vi "GT Helix ZXCY.vi"(0 "cardNum":i16, 1 "crd":i16, 2 "x":i32, 3 "y":i32, 4 "z":i32, 5 "zCenter":dbl, 6 "xCenter":dbl, 7 "error in (no error)":errorcluster caption="错误输入（无错误）", 8 "circleDir":i16, 9 "synVel":dbl, 10 "synAcc":dbl, 11 "velEnd":dbl, 12 "fifo":i16) -> (20 "function return":i16, 27 "error out":errorcluster caption="错误输出")   [LabVIEW 2014, in "gts.lvlib"]
doc: "GT_API GT_HelixZXCY(short cardNum,short crd,long x,long y,long z,double zCenter,double xCenter,short circleDir,double synVel,double synAcc,double velEnd=0,short fifo=0);"
uses:
  gts.lvlib
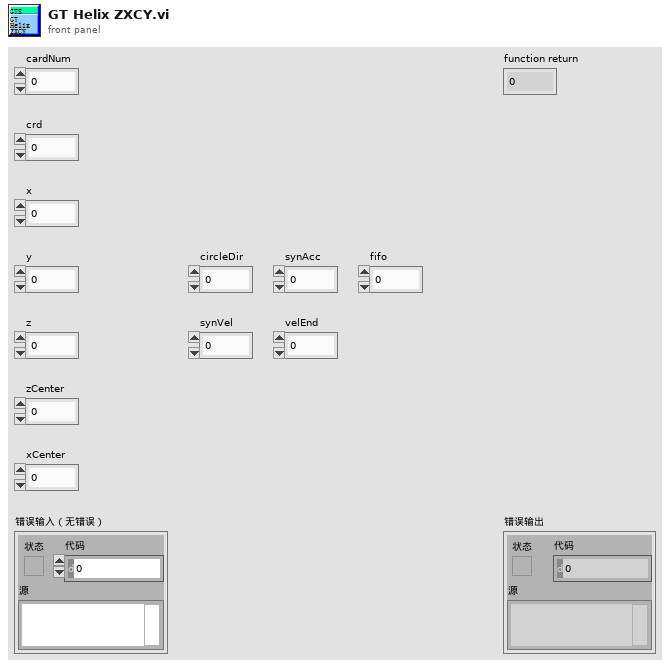
[diagram p1: front panel]
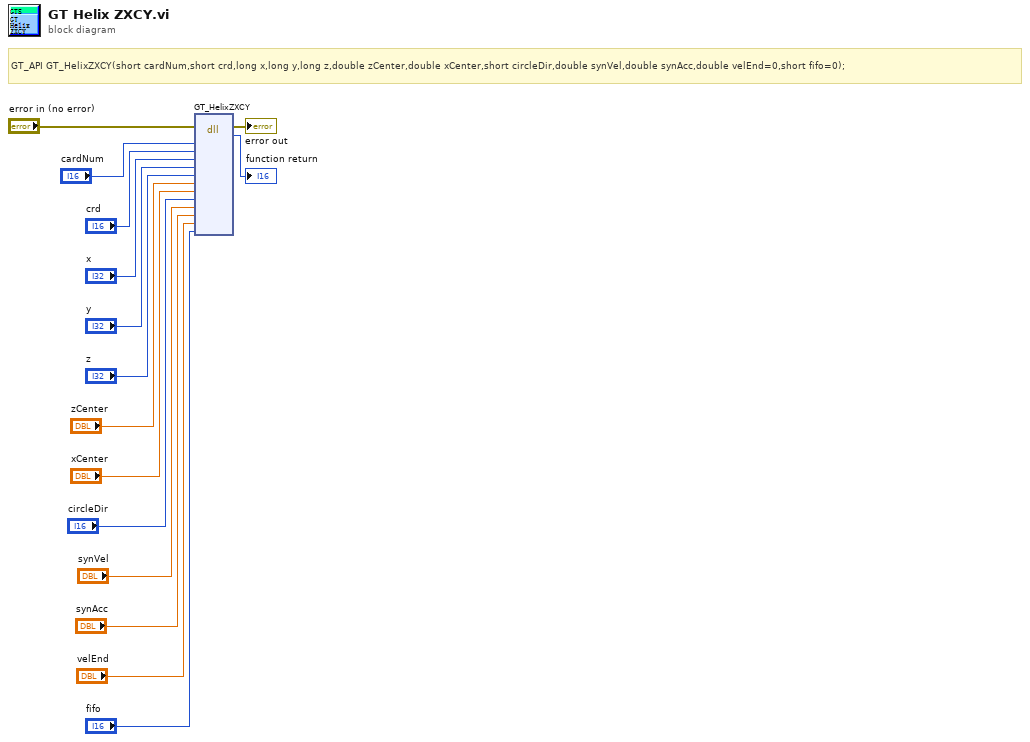
[diagram p0: block diagram]
diagram:
  # "GT_API GT_HelixZXCY(short cardNum,short crd,long x,long y,long z,double zCenter,double xCenter,short circleDir,double synVel,double synAcc,double velEnd=0,short fifo=0);"
  n1 = dll-call lib="PTH2habs D固高科技资料GTS控制卡GTS卡18年上半年资料dllVC32bit\nmulti_cardgts.*" fn="GT_HelixZXCY"(error in="error in (no error)", "cardNum"="cardNum", "crd"="crd", "x"="x", "y"="y", "z"="z", "zCenter"="zCenter", "xCenter"="xCenter", "circleDir"="circleDir", "synVel"="synVel", "synAcc"="synAcc", "velEnd"="velEnd", "fifo"="fifo") -> (error out=→"error out":errorcluster, →"function return":i16)  [unwired: 14 in, 1 out]
